vi "applicationStop.vi"(8 "error in":errorcluster, 9 "Boiler Simulation Controls":refnum<vi>, 10 "Boiler Controls":refnum<vi>, 11 "Boiler Status Indicators":refnum<vi>) -> (0 "error out":errorcluster)   [LabVIEW 2024]
uses:
  Controls/Boiler Simulation Controls.ctl
  Controls/Boiler Status Indicators.ctl
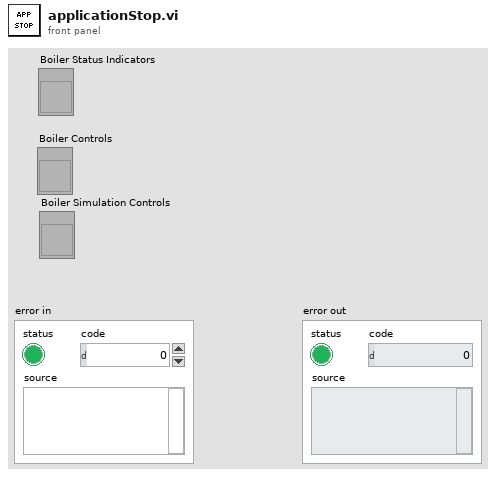
[diagram p1: front panel]
types:
  T1 = typedef "Boiler Status Indicators.ctl" = cluster{"Status":string, "Primary Fan":bool, "Natural Gas Valve":bool, "Pilot":bool, "Fuel Valve":bool, "Forced Draft Fan":bool, "Time Count":dbl}
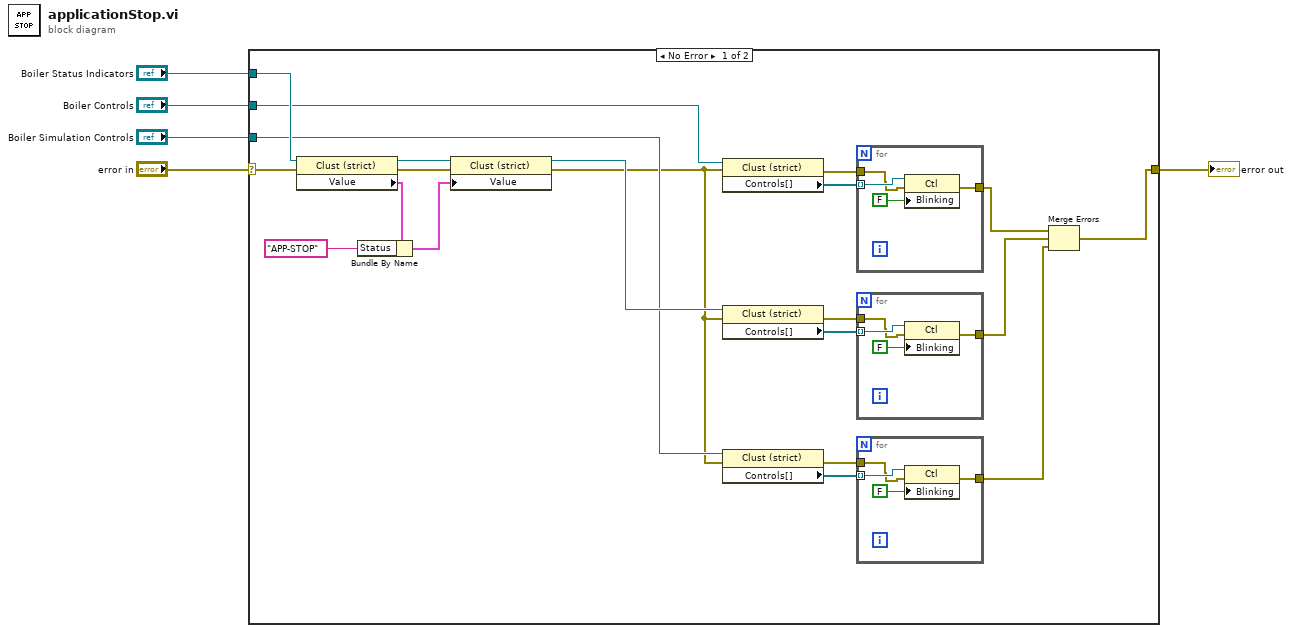
[diagram p0: block diagram]
diagram:
  n1 = case shown="No Error" "error in" {
    selector: "error in" -> [w26 w39]
    tunnel: [w6 w39] -> w4
    tunnel: "Boiler Status Indicators" -> [w25 _]
    tunnel: "Boiler Controls" -> [w19 _]
    tunnel: "Boiler Simulation Controls" -> [w14 _]
    frame No Error {
      n2 = property class="Clust (strict)"(reference=w25, error in=w26) -> (reference out=w24:refnum<vi>, error out=w23:errorcluster, "Value"=w22:T1)
      n3 = Bundle By Name(cluster=w22, "Status"="APP-STOP") -> (w21:T1)
      n4 = property class="Clust (strict)"(reference=w24, error in=w23, "Value"=w21) -> (reference out=w15:refnum<vi>, error out=w13:errorcluster)
      n5 = property class="Clust (strict)"(reference=w19, error in=w13) -> (error out=w12:errorcluster, "Controls[]"=w18:refnum<vi>[])  [unwired: 1 out]
      n6 = property class="Clust (strict)"(reference=w15, error in=w13) -> (error out=w11:errorcluster, "Controls[]"=w17:refnum<vi>[])  [unwired: 1 out]
      n7 = property class="Clust (strict)"(reference=w14, error in=w13) -> (error out=w10:errorcluster, "Controls[]"=w16:refnum<vi>[])  [unwired: 1 out]
      n8 = for {
        tunnel: w18 -> [w38] mode=indexing
        tunnel: w12 -> [w36]
        tunnel: [w35] -> w9
        n9 = property class="Ctl"(reference=w38, error in=w36, "Blinking"=FALSE) -> (error out=w35:errorcluster)  [unwired: 1 out]
      }
      n10 = for {
        tunnel: w17 -> [w34] mode=indexing
        tunnel: w11 -> [w32]
        tunnel: [w31] -> w8
        n11 = property class="Ctl"(reference=w34, error in=w32, "Blinking"=FALSE) -> (error out=w31:errorcluster)  [unwired: 1 out]
      }
      n12 = for {
        tunnel: w16 -> [w30] mode=indexing
        tunnel: w10 -> [w28]
        tunnel: [w27] -> w7
        n13 = property class="Ctl"(reference=w30, error in=w28, "Blinking"=FALSE) -> (error out=w27:errorcluster)  [unwired: 1 out]
      }
      n14 = Merge Errors(w9, w8, w7) -> (w6:errorcluster)
    }
    frame Error {
    }
  }
  "error out" <- w4
